vi "FPGA_DIOWriteSlowValueRelayFwd.vi"(8 "error in (no error)":errorcluster, 10 "Relay Forward":u8, 11 "DIODeviceRef In":T1) -> (0 "error out":errorcluster, 3 "DIODeviceRef Out":T1)   [LabVIEW 2017]
uses:
  <vilib>/Rock Robotics/SystemInterfaces/DIO/FPGA_DIODevRef.ctl
  <vilib>/Rock Robotics/SystemInterfaces/System/FPGA_SystemFPGA Ref Global.vi
  <vilib>/Utility/error.llb/Error Cluster From Error Code.vi
  <vilib>/rvi/errors/niLvFpgaAdjustHostInterfaceError.vi
  <vilib>/rvi/interface/nirviReadWriteControl/nirviReadWriteControl.xnode
  <vilib>/Rock Robotics/SystemInterfaces/System/FPGA_SystemFRC FPGA Ref.ctl
  <vilib>/rvi/interface/Simulation/niFpgaSimulationCallBeginRW.vi
  NiFpgaLv.dll
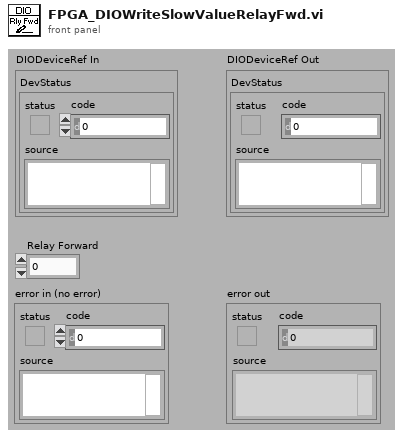
[diagram p1: front panel]
types:
  T1 = typedef "FPGA_DIODevRef.ctl" = cluster{"DevStatus":errorcluster}
  T2 = typedef "FPGA_SystemFRC FPGA Ref.ctl" = refnum<k20>
  T3 = cluster{"Forward":fxp<+,4,4>, "Reverse":fxp<+,4,4>}
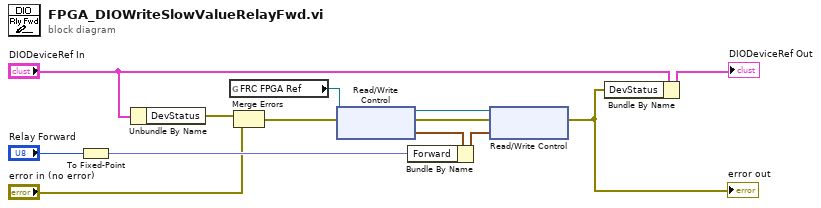
[diagram p0: block diagram]
diagram:
  n1 = To Fixed-Point(number="Relay Forward") -> (fixed-point=w7:fxp<+,4,4>)  [unwired: 1 in]
  n2 = Unbundle By Name("DIODeviceRef In") -> ("DevStatus"=w9:errorcluster)
  n3 = global read "FPGA_SystemFPGA Ref Global.vi" "FRC FPGA Ref"() -> (w1:T2)
  n4 = Merge Errors(w9, "error in (no error)") -> (w8:errorcluster)
  n5 = xnode "Read/Write Control"("FPGA VI Reference In"=w1, "error in"=w8) -> ("FPGA VI Reference Out"=w6:T2, "error out"=w5:errorcluster, "Relay.Value"=w4:T3)
  n6 = Bundle By Name(cluster=w4, "Forward"=w7) -> (w3:T3)
  n7 = xnode "Read/Write Control"("FPGA VI Reference In"=w6, "error in"=w5, "Relay.Value"=w3) -> ("error out"=w10:errorcluster)  [unwired: 1 out]
  "error out" <- w10
  n8 = Bundle By Name(cluster="DIODeviceRef In", "DevStatus"=w10) -> (→"DIODeviceRef Out":T1)
